vi "PH_Periodic_Sequencer.ProcEvents.vi"(0 "i ref in":refnum<vi>, 5 "error in (no error)":errorcluster) -> (14 "i ref out":refnum<vi>, 19 "error out":errorcluster)   [LabVIEW 2014, in "PH_Periodic_Sequencer.lvlib"]
doc: "This method is used to define the events the object will listen to. Add your own events here."
uses:
  PH_Periodic_Sequencer.lvlib
  CSCore/BaseProcess/BaseProcess.event definition.ctl
  CSCore/CAEObj/CAEObj.event definition.ctl
  CSCore/BaseProcess/BaseProcess.descriptor string definition.ctl
  CSCore/BaseProcess/BaseProcess.lvlib
  CSCore/CAEObj/CAEObj.lvlib
  PH_Common/PH_Common.lvlib
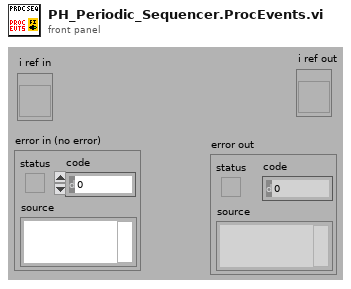
[diagram p1: front panel]
types:
  T1 = typedef "BaseProcess.lvlib/BaseProcess.event definition.ctl" = cluster{"CAEEvtDef":T2, "Data Descriptor":T3}
  T2 = typedef "CAEObj.lvlib/CAEObj.event definition.ctl" = cluster{"URL":string, "enable":bool, "ignoreResID":bool}
  T3 = typedef "BaseProcess.lvlib/BaseProcess.descriptor string definition.ctl" = string
  T4 = typedef "PH_Periodic_Sequencer.lvlib/PH_Periodic_Sequencer.i attribute.ctl" = cluster{"GUI Refs":cluster{"Main Off":refnum<vi>, "Start":refnum<vi>, "Ready":refnum<vi>, "Sequencer SM State":refnum<vi>, "Interval [sec]":refnum<vi>, "Wanted Shots":refnum<vi>, "Delivered Shots":refnum<vi>}, "PU Info":cluster{"Instancename":string, "State":T5, "linked":bool}[], "Sequencer":cluster{"Instancename":string, "linked?":bool, "R2S?":bool, "SM State":string}, "Run?":bool, "Interval [sec]":dbl, "PU State Refs":refnum<vi>[], "Wanted Shots":i32, "Delivered Shots":i32}
  T5 = typedef "PH_StatusHandler.lvlib/PH_StatusHandler.Status.ctl" = i16
  T6 = cluster{"Instancename":string, "State":T5, "linked":bool}[]
  T7 = typedef "PH_Common.lvlib/PH_DIM.Event Declarer.ctl" = cluster{"Service Name":string, "Selector":string}
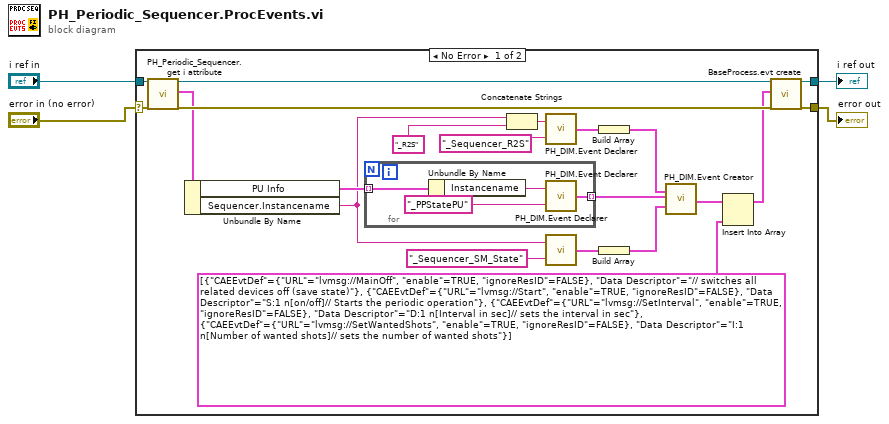
[diagram p0: block diagram]
diagram:
  n1 = case shown="No Error" "error in (no error)" {
    selector: "error in (no error)" -> [w17 w30]
    tunnel: "i ref in" -> [w22 w31]
    tunnel: [w21 w31] -> w3
    tunnel: [w20 w30] -> w2
    frame No Error {
      n2 = call "PH_Periodic_Sequencer.get i attribute.vi"("i ref in"=w22, "error in (no error)"=w17) -> ("i ref out"=w25:refnum<vi>, "i attribute"=w16:T4, "error out"=w24:errorcluster)  [unwired: 15 in]
      n3 = Unbundle By Name(w16) -> ("PU Info"=w13:T6, "Sequencer.Instancename"=w10:string)
      n4 = for {
        tunnel: [w29] -> w14 mode=indexing
        tunnel: w13 -> [w27] mode=indexing
        n5 = Unbundle By Name(w27) -> ("Instancename"=w26:string)
        n6 = call "PH_DIM.Event Declarer.vi"("Selector"="_PPStatePU" ("URL"), "Service Name"=w26) -> ("declared DIM Event"=w29:T7)
      }
      n7 = Concatenate Strings(w10, "_R2S" ("string")) -> (w6:string)
      n8 = call "PH_DIM.Event Declarer.vi"("Selector"="_Sequencer_R2S" ("URL"), "Service Name"=w6) -> ("declared DIM Event"=w7:T7)
      n9 = call "PH_DIM.Event Declarer.vi"("Selector"="_Sequencer_SM_State" ("URL"), "Service Name"=w10) -> ("declared DIM Event"=w11:T7)
      n10 = Build Array(w7) -> (w8:T7[])
      n11 = Build Array(w11) -> (w12:T7[])
      n12 = call "PH_DIM.Event Creator.vi"("Trendmessage Services"=w8, "Status Services"=w14, "SM State Services"=w12) -> ("DIM Service Events"=w18:T1[])  [unwired: 16 in]
      n13 = Insert Into Array(array=w18, new element=T1[] [{"CAEEvtDef"={"URL"="lvmsg://MainOff", "enable"=TRUE, "ignoreResID"=FALSE}, "Data Descriptor"="// switches all related devices off (save state)"}, {"CAEEvtDef"={"URL"="lvmsg://Start", "enable"=TRUE, "ignoreResID"=FALSE}, "Data Descriptor"="S:1 n[on/off]// Starts the periodic operation"}, {"CAEEvtDef"={"URL"="lvmsg://SetInterval", "enable"=TRUE, "ignoreResID"=FALSE}, "Data Descriptor"="D:1 n[Interval in sec]// sets the interval in sec"}, {"CAEEvtDef"={"URL"="lvmsg://SetWantedShots", "enable"=TRUE, "ignoreResID"=FALSE}, "Data Descriptor"="I:1 n[Number of wanted shots]// sets the number of wanted shots"}] ("new events")) -> (w23:T1[])  [unwired: 1 in]
      n14 = call "BaseProcess.evt create.vi"("i ref in"=w25, "newEvents"=w23, "error in (no error)"=w24) -> ("i ref out"=w21:refnum<vi>, "error out"=w20:errorcluster)  [unwired: 13 in, 2 out]
    }
    frame Error {
    }
  }
  "i ref out" <- w3
  "error out" <- w2
